vi "Autonomous Vehicle Simulation.vi"(4 "Direction":bool=TRUE, 5 "Brake":bool, 6 "Steering":dbl(slide) min=-1.0 max=1.0 step=1e-05 scale=-1.0..1.0) -> (0 "error out":errorcluster, 1 "fps":dbl, 2 "Map":picture, 3 "Camera":picture)   [LabVIEW 2025]
doc: "Enables users to control the vehicle's steering, throttle, brakes, starting position, and weather simulation in real time.\n\n*This is a free driving scenario with other vehicles spawning on specified positions in autopilot mode*"
panel:
  in  "Throttle":dbl(slide) scale=0.0..1.0
  in  "Vehicle Start Position":i32=1 min=-1 max=2 step=1
  in  "stop":bool
  out "Weather Profiles":T1(array[cluster])
  # "Steering"
  # "FPS"
  # "Apply Brakes"
  # "Direction"
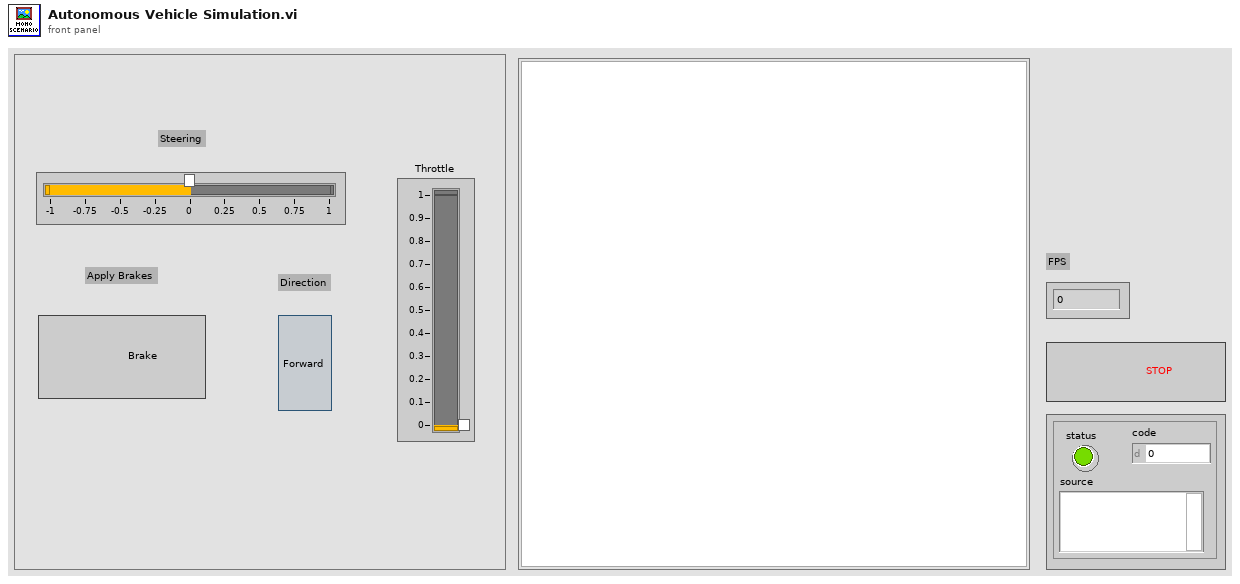
[diagram p1: front panel]
types:
  T1 = cluster{"id":string, "CloudColor":cluster{"A":sgl, "B":sgl, "G":sgl, "R":sgl}, "CloudOpacity":sgl, "Day":sgl, "FogCutoffDistance":sgl, "FogDensity":sgl, "FogHeightFalloff":sgl, "FogInscatteringColor":cluster{"A":sgl, "B":sgl, "G":sgl, "R":sgl}, "FogMaxOpacity":sgl, "FogStartDistance":sgl, "HorizonColor":cluster{"A":sgl, "B":sgl, "G":sgl, "R":sgl}, "HorizonFalloff":sgl, "Hours":sgl, "IsDaylightSavingTime":bool, "Latitude":sgl, "Longitude":sgl, "Minutes":sgl, "Month":sgl, "NorthOffset":sgl, "OverallSkyColor":cluster{"A":sgl, "B":sgl, "G":sgl, "R":sgl}, "OverideTimeBasedSunAngle":bool, "PrecipitationAccumulation":sgl, "PrecipitationAmount":sgl, "PrecipitationType":string, "SecondFogDensity":sgl, "SecondFogHeightFalloff":sgl, "SecondFogHeightOffset":sgl, "Seconds":sgl, "SkyLightColor":cluster{"A":sgl, "B":sgl, "G":sgl, "R":sgl}, "SkyLightIntensity":sgl, "StarBrightness":sgl, "SunAzimuthAngle":sgl, "SunBrightness":sgl, "SunDirectionalLightColor":cluster{"A":sgl, "B":sgl, "G":sgl, "R":sgl}, "SunDirectionalLightIntensity":sgl, "SunPolarAngle":sgl, "TimeZone":sgl, "WindAngle":sgl, "WindIntensity":sgl, "Year":sgl, "ZenithColor":cluster{"A":sgl, "B":sgl, "G":sgl, "R":sgl}, "bPrecipitation":bool, "bWind":bool}[]
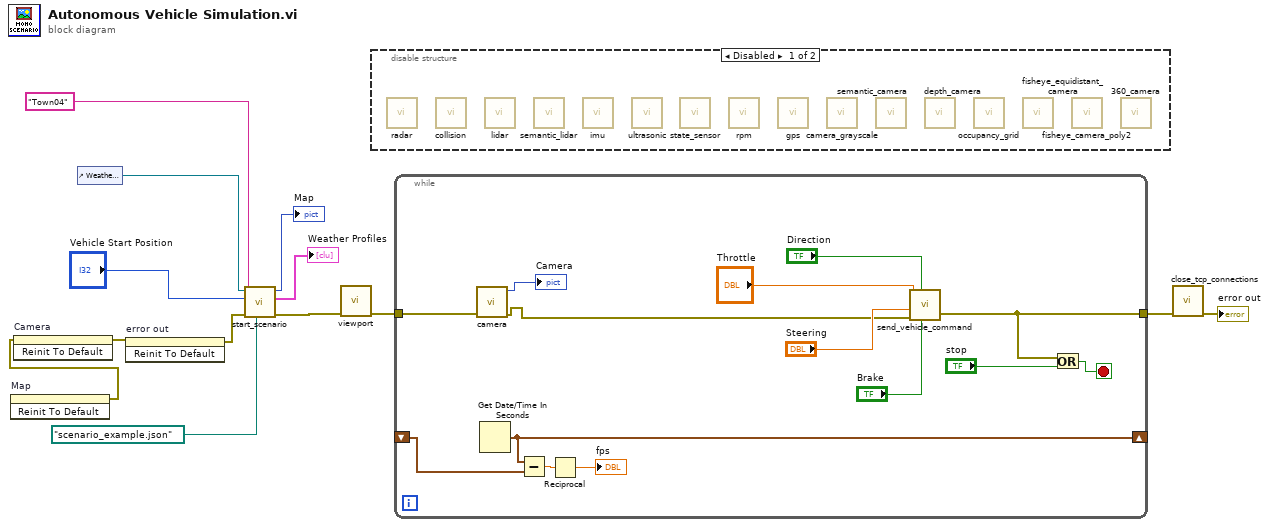
[diagram p0: block diagram]
diagram:
  n1 = invoke on="Map" class="Pict" method="Reinit To Default"() -> (error out=w8:errorcluster)  [unwired: 3 in, 2 out]
  n2 = invoke on="Camera" class="Pict" method="Reinit To Default"(error in=w8) -> (error out=w9:errorcluster)  [unwired: 2 in, 2 out]
  n3 = control-ref of="Weather Profiles"() -> (w1:refnum<vi>)
  n4 = invoke on="error out" class="Clust (strict)" method="Reinit To Default"(error in=w9) -> (error out=w13:errorcluster)  [unwired: 2 in, 2 out]
  n5 = call "start_scenario.vi"("Scenario Configuration"=path "scenario_example.json", "error in"=w13, "Select a map"="Town04", "Vehicle Start Position"="Vehicle Start Position", "Weather Profiles"=w1) -> ("error out"=w12:errorcluster, "Weather Profiles"=→"Weather Profiles":T1, "Map"=→"Map":picture)  [unwired: 2 in]
  n6 = call "viewport.vi"("Error In"=w12) -> ("Error Out"=w11:errorcluster)  [unwired: 6 in]
  n7 = disable-structure shown="Disabled" {
    frame Disabled {
      n8 = call "radar.vi"() -> ()  [unwired: 4 in, 5 out]
      n9 = call "collision.vi"() -> ()  [unwired: 4 in, 4 out]
      n10 = call "lidar.vi"() -> ()  [unwired: 4 in, 4 out]
      n11 = call "semantic_lidar.vi"() -> ()  [unwired: 4 in, 4 out]
      n12 = call "imu.vi"() -> ()  [unwired: 4 in, 4 out]
      n13 = call "ultrasonic.vi"() -> ()  [unwired: 3 in, 4 out]
      n14 = call "state_sensor.vi"() -> ()  [unwired: 4 in, 4 out]
      n15 = call "rpm.vi"() -> ()  [unwired: 4 in, 4 out]
      n16 = call "gps.vi"() -> ()  [unwired: 4 in, 4 out]
      n17 = call "camera_grayscale.vi"() -> ()  [unwired: 5 in, 5 out]
      n18 = call "semantic_camera.vi"() -> ()  [unwired: 5 in, 5 out]
      n19 = call "depth_camera.vi"() -> ()  [unwired: 5 in, 5 out]
      n20 = call "occupancy_grid.vi"() -> ()  [unwired: 5 in, 5 out]
      n21 = call "fisheye_equidistant_camera.vi"() -> ()  [unwired: 5 in, 4 out]
      n22 = call "fisheye_camera_poly2.vi"() -> ()  [unwired: 5 in, 4 out]
      n23 = call "360_camera.vi"() -> ()  [unwired: 5 in, 4 out]
    }
    frame Enabled {
    }
  }
  n24 = while {
    shift-right: [w27] -> _
    shift-left: _ -> [w26]
    tunnel: w11 -> [w15]
    tunnel: [w23] -> w7
    stop <- w24 stop-if-true
    n25 = call "camera.vi"("error In"=w15) -> ("Image"=→"Camera":picture, "error out"=w16:errorcluster)  [unwired: 4 in, 3 out]
    n26 = Get Date/Time In Seconds() -> (seconds since 1Jan1904=w27:timestamp)
    n27 = Subtract(x=w27, y=w26) -> (x-y=w25:dbl)
    n28 = Reciprocal(x=w25) -> (1/x=→"fps":dbl)
    n29 = call "send_vehicle_command.vi"("Brake"="Brake", "Drive mode"="Direction", "error in"=w16, "Right amount"="Steering", "Forward amount"="Throttle") -> ("error out"=w23:errorcluster)  [unwired: 2 in]
    n30 = Or(x=w23, y="stop") -> (x .or. y?=w24:bool)
  }
  n31 = call "close_tcp_connections.vi"("error in"=w7) -> ("error out"=→"error out":errorcluster)  [unwired: 6 in]
